vi "Configure Temperature.vi"(0 "VISA resource name":refnum<visa-resource-name>, 1 "Function":i32(ring) items=["Primary", "Secondary"], 3 "Temperature Units (0: Celsius)":u16(ring) items=["Celsius", "Fahrenheit", "Kelvin"], 5 "error in (no error)":errorcluster, 6 "RTD Type  (PT100)":u16(ring) items=["PT100", "D100", "F100", "PT385", "PT3916", "User-Defined", "SPRTD", "NTCT"], 7 "Digital Filter (0: Off)":u16(ring) items=["Off", "Moving Filter", "Repeating Filter"], 8 "User-Defined":T2={"R-Zero"=100.0, "Alpha"=0.00385, "Beta"=0.10863, "Delta"=1.4999}, 9 "Digital Filter Readings (10)":i32=10, 10 "Standard Platinum RTD":T1={"R-Zero"=100.0, "A4"=0.0, "B4"=0.0, "AX"=0.0, "BX"=0.0, "CX"=0.0, "DX"=0.0}, 11 "NTCT":cluster{"A":dbl, "C":dbl, "B":dbl}={"A"=0.001129241, "C"=8.77546e-08, "B"=0.0002341077} {"B" format="%#_10g"; "C" format="%#_12g"; "A" format="%#_10g"}) -> (14 "VISA resource name out":refnum<visa-resource-name>, 19 "error out":errorcluster)   [LabVIEW 2020, in "Keithley 2100 Series.lvlib"]
doc: "This VI configures the instrument to measure temperature.\n\nNotes:\nThe multimeter supports both thermocouple and RTD. User needs to configure the multimeter for the right sensor type before they can make temperature measurements.\n\nRTD Definition:\n\nIf you are using RTD, the options are: PT100, D100, F100, PT385, PT3916, user-defined RTD, NTCT and SPRTD. If you need to change the factors that are used to calculate the temperature in RTD, choose user-defined RTD in which you are able to change any factors as you wish."
uses:
  Keithley 2100 Series.lvlib
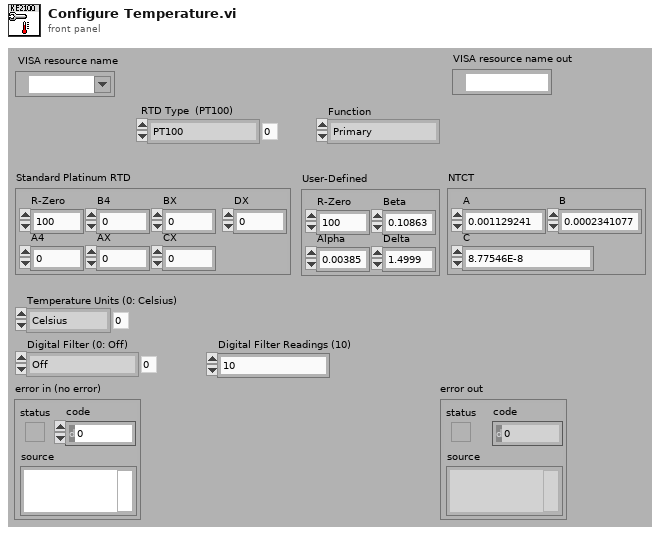
[diagram p1: front panel]
types:
  T1 = cluster{"R-Zero":dbl, "A4":dbl, "B4":dbl, "AX":dbl, "BX":dbl, "CX":dbl, "DX":dbl}
  T2 = cluster{"R-Zero":dbl, "Alpha":dbl, "Beta":dbl, "Delta":dbl}
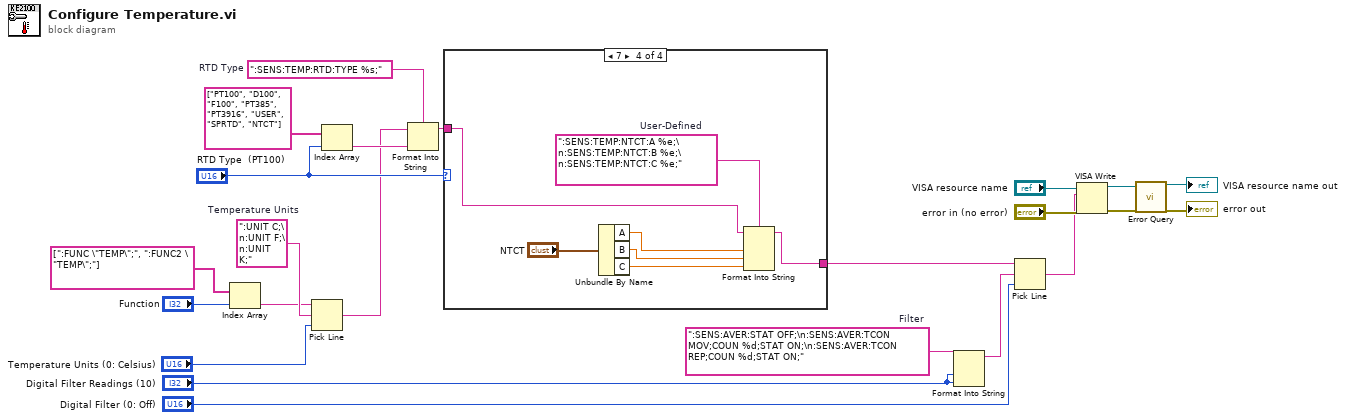
[diagram p0: block diagram]
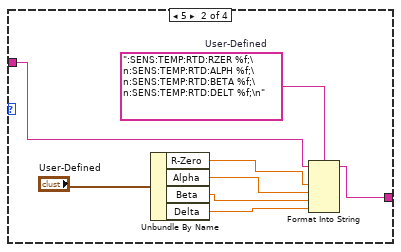
[diagram p3: hidden frame]
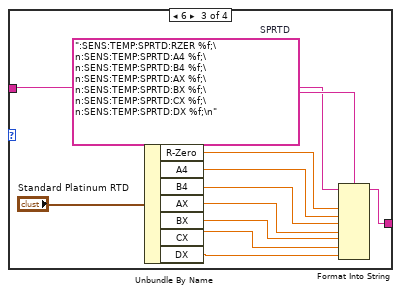
[diagram p4: hidden frame]
diagram:
  w10 = ":SENS:TEMP:RTD:TYPE %s;"  # RTD Type
  w15 = ":UNIT C;\n:UNIT F;\n:UNIT K;"  # Temperature Units
  w21 = ":SENS:AVER:STAT OFF;\n:SENS:AVER:TCON MOV;COUN %d;STAT ON;\n:SENS:AVER:TCON REP;COUN %d;STAT ON;"  # Filter
  n1 = Index Array(array=string[] [":FUNC \"TEMP\";", ":FUNC2 \"TEMP\";"], index="Function") -> (element=w1:string)
  n2 = Pick Line(string ("")=w1, multi-line string=w15, line index="Temperature Units (0: Celsius)") -> (output string=w6:string)
  n3 = Index Array(array=string[] ["PT100", "D100", "F100", "PT385", "PT3916", "USER", "SPRTD", "NTCT"], index="RTD Type  (PT100)") -> (element=w9:string)
  n4 = Format Into String(format string=w10, initial string=w6, w9) -> (resulting string=w7:string)  [unwired: 1 in, 1 out]
  n5 = case shown="7" "RTD Type  (PT100)" {
    tunnel: w7 -> [w24 w25 w33 w45]
    tunnel: [w24 w26 w41 w46] -> w5
    frame 0, Default {
    }
    frame 5 {
      w27 = ":SENS:TEMP:RTD:RZER %f;\n:SENS:TEMP:RTD:ALPH %f;\n:SENS:TEMP:RTD:BETA %f;\n:SENS:TEMP:RTD:DELT %f;\n"  # User-Defined
      n6 = Unbundle By Name("User-Defined") -> ("R-Zero"=w31:dbl, "Alpha"=w30:dbl, "Beta"=w29:dbl, "Delta"=w28:dbl)
      n7 = Format Into String(format string=w27, initial string=w25, w31, w30, w29, w28) -> (resulting string=w26:string)  [unwired: 1 in, 1 out]
    }
    frame 6 {
      w42 = ":SENS:TEMP:SPRTD:RZER %f;\n:SENS:TEMP:SPRTD:A4 %f;\n:SENS:TEMP:SPRTD:B4 %f;\n:SENS:TEMP:SPRTD:AX %f;\n:SENS:TEMP:SPRTD:BX %f;\n:SENS:TEMP:SPRTD:CX %f;\n:SENS:TEMP:SPRTD:DX %f;\n"  # SPRTD
      n8 = Unbundle By Name("Standard Platinum RTD") -> ("R-Zero"=w40:dbl, "A4"=w39:dbl, "B4"=w38:dbl, "AX"=w37:dbl, "BX"=w36:dbl, "CX"=w35:dbl, "DX"=w34:dbl)
      n9 = Format Into String(format string=w42, initial string=w33, w40, w39, w38, w37, w36, w35, w34) -> (resulting string=w41:string)  [unwired: 1 in, 1 out]
    }
    frame 7 {
      w47 = ":SENS:TEMP:NTCT:A %e;\n:SENS:TEMP:NTCT:B %e;\n:SENS:TEMP:NTCT:C %e;"  # User-Defined
      n10 = Unbundle By Name("NTCT") -> ("A"=w50:dbl, "B"=w49:dbl, "C"=w48:dbl)
      n11 = Format Into String(format string=w47, initial string=w45, w50, w49, w48) -> (resulting string=w46:string)  [unwired: 1 in, 1 out]
    }
  }
  n12 = Format Into String(format string=w21, "Digital Filter Readings (10)", "Digital Filter Readings (10)") -> (resulting string=w22:string)  [unwired: 2 in, 1 out]
  n13 = Pick Line(string ("")=w5, multi-line string=w22, line index="Digital Filter (0: Off)") -> (output string=w4:string)
  n14 = VISA Write(VISA resource name="VISA resource name", write buffer=w4, error in (no error)="error in (no error)") -> (VISA resource name out=w17:refnum<visa-resource-name>, error out=w16:errorcluster)  [unwired: 1 out]
  n15 = call "Error Query.vi"("VISA resource name"=w17, "error in (no error)"=w16) -> ("VISA resource name out"=→"VISA resource name out":refnum<visa-resource-name>, "error out"=→"error out":errorcluster)  [unwired: 14 in, 2 out]
